vi "AudioOUT.vi"   [LabVIEW 2016]
uses:
  Global 1.vi
  <vilib>/rvi/eio/common/nirviEmuTemplateMethod_errors.vi
  <vilib>/eio/EIONode/EIONode.xnode
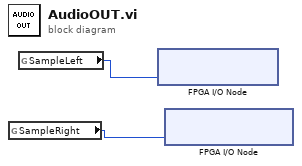
[diagram p0: block diagram]
diagram:
  n1 = global read "Global 1.vi" "SampleRight"() -> (w1:i16)
  n2 = global read "Global 1.vi" "SampleLeft"() -> (w2:i16)
  n3 = xnode "FPGA I/O Node"("AudioOut/Left"=w2) -> ()  [unwired: 1 in, 1 out]
  n4 = xnode "FPGA I/O Node"("AudioOut/Right"=w1) -> ()  [unwired: 1 in, 1 out]
